vi "2_Medir_Temperatura.vi"() -> ()   [LabVIEW 2020]
panel:
  in  "Tiempo de espera":dbl(slide) scale=0.0..1000.0
  out "Thermometer":dbl(slide) scale=0.0..50.0
  out "Waveform Chart":dynamicdata(graph)
  out "Temperatura":dbl
  in  "stop":bool
  out "Voltaje":dbl
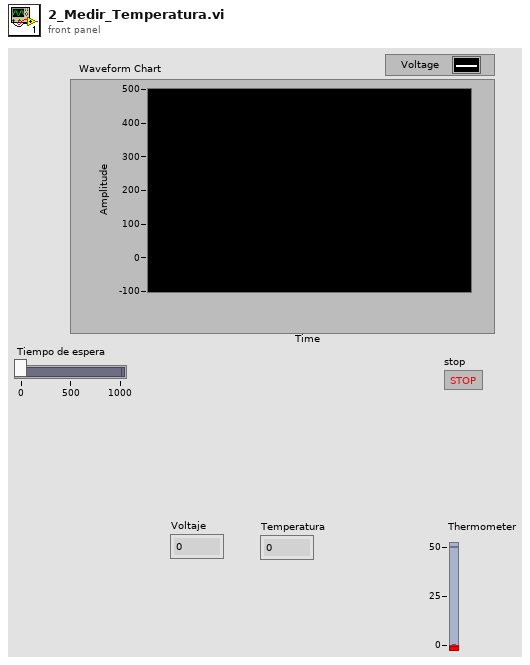
[diagram p1: front panel]
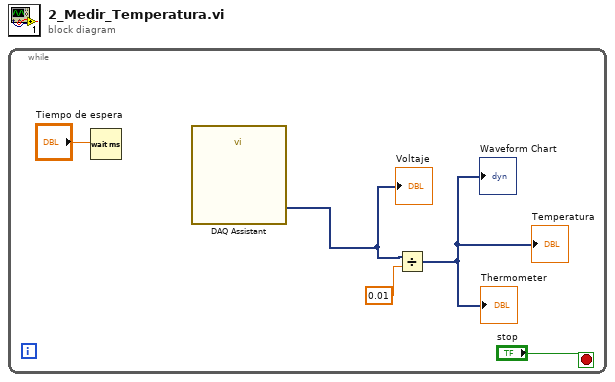
[diagram p0: block diagram]
diagram:
  n1 = while {
    stop <- "stop" stop-if-true
    n2 = Wait (ms)(milliseconds to wait="Tiempo de espera") -> ()  [unwired: 1 out]
    n3 = call "DAQ Assistant"() -> ("data"=w1:dynamicdata)  [unwired: 17 in, 2 out]
    "Voltaje" <- w1
    n4 = Divide(x=w1, y=0.01) -> (x/y=→"Thermometer" →"Waveform Chart" →"Temperatura":dynamicdata)
  }
